vi "Update Check-in Status.vi"(0 "Guest Manager Model in":refnum<class "Guest Manager Model.lvclass">, 5 "IsSuccess":bool, 7 "Reason If Failure":string, 11 "error in (no error)":errorcluster) -> (4 "Guest Manager Model out":refnum<class "Guest Manager Model.lvclass">, 15 "error out":errorcluster)   [LabVIEW 2023, in "Guest Manager Model.lvlib" / "Guest Manager Model.lvclass"]
uses:
  Guest Manager Model.lvclass
  Guest Manager Model.lvclass/Guest Manager Model.ctl
  Guest Manager UI/Guest Manager UI Messages/Update Guest Name Msg/Update Guest Name Msg.lvclass/Update Guest Name Msg.ctl
  <vilib>/ActorFramework/Message Enqueuer/Message Enqueuer.lvclass/Message Enqueuer.ctl
  <vilib>/ActorFramework/Message Enqueuer/Enqueue.vi
  Guest Manager UI/Guest Manager UI Messages/Update Guest Name Msg/Update Guest Name Msg.lvclass
  C:/Program Files/National Instruments/LabVIEW 2023/vi.lib/ActorFramework/Message/Message.lvclass
  <vilib>/ActorFramework/Message Priority Queue/Priority Enqueue.vi
  Guest Manager UI/Guest Manager UI Messages/Update Check-in Status Msg/Update Check-in Status Msg.lvclass
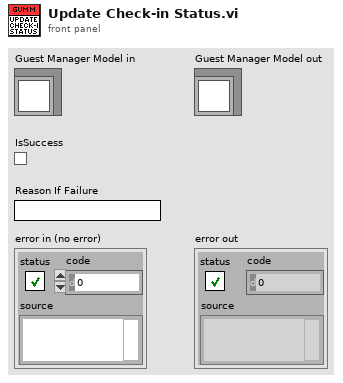
[diagram p1: front panel]
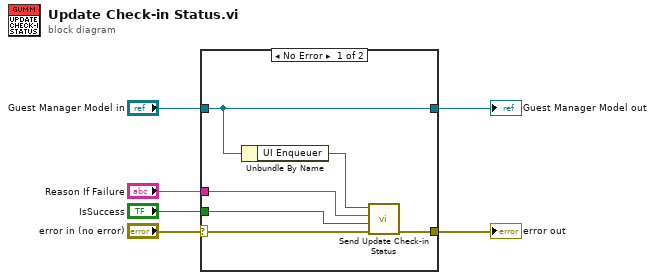
[diagram p0: block diagram]
diagram:
  n1 = case shown="No Error" "error in (no error)" {
    selector: "error in (no error)" -> [w12 w14]
    tunnel: [w11 w14] -> w5
    tunnel: [w8 w13] -> w3
    tunnel: "Guest Manager Model in" -> [w8 w13]
    tunnel: "Reason If Failure" -> [w10 _]
    tunnel: "IsSuccess" -> [w9 _]
    frame No Error {
      n2 = Unbundle By Name(w8) -> ("UI Enqueuer"=w7:refnum<class "Message Enqueuer.lvclass">)
      n3 = call "Send Update Check-in Status.vi"("error in (no error)"=w12, "IsSuccess"=w9, "Reason If Failure"=w10, "Message Enqueuer"=w7) -> ("error out"=w11:errorcluster)  [unwired: 6 in, 1 out]
    }
    frame Error {
    }
  }
  "error out" <- w5
  "Guest Manager Model out" <- w3
